vi "DaNISim.vi"(4 "Sonar offset angle":dbl, 5 "Action":enum16{"Init", "Run", "Release"}(ring), 6 "Sonar angle":dbl, 7 "Mode Select":T1(ring), 8 "error in (no error)":errorcluster, 9 "IP Adress":T2, 10 "Ul":dbl, 11 "Ur":dbl) -> (0 "error out":errorcluster, 1 "Sonar distance":fxp<+,32,8>, 2 "OmegaL":dbl, 3 "OmegaR":dbl)   [LabVIEW 2016]
uses:
  <vilib>/userdefined/High Color/nirio_resource_hc.ctl
  <vilib>/FPGAPlugInAG/sbRIO-9632/niLvFpga_Open_sbRIO-9632.vi
  <vilib>/rvi/interface/common/dynamic/niFpgaDynamicAddResources.vi
  <vilib>/Utility/error.llb/Error Cluster From Error Code.vi
  <vilib>/rvi/errors/niLvFpgaAdjustHostInterfaceError.vi
  <vilib>/FPGAPlugInAG/Dynamic/niLvFpga_Close_Dynamic.vi
  <vilib>/rvi/interface/nirviOpenFPGA/nirviOpenFPGA.xnode
  FPGA Bitfiles/StarterKit2.0Cus_FPGATarget_StarterKit2.0Cus_pLn805qeh78.lvbitx
  <vilib>/rvi/interface/nirviReadWriteControl/nirviReadWriteControl.xnode
  <vilib>/rvi/interface/nirviCloseFPGA/nirviCloseFPGA.xnode
  NiFpgaLv.dll
  <vilib>/rvi/interface/Simulation/niFpgaSimulationCallBeginRW.vi
panel:
  in  "N":i32=100
  in  "J":dbl=0.03
  in  "L":dbl=0.1825
  in  "R":dbl=0.046
  in  "M":dbl=3.0
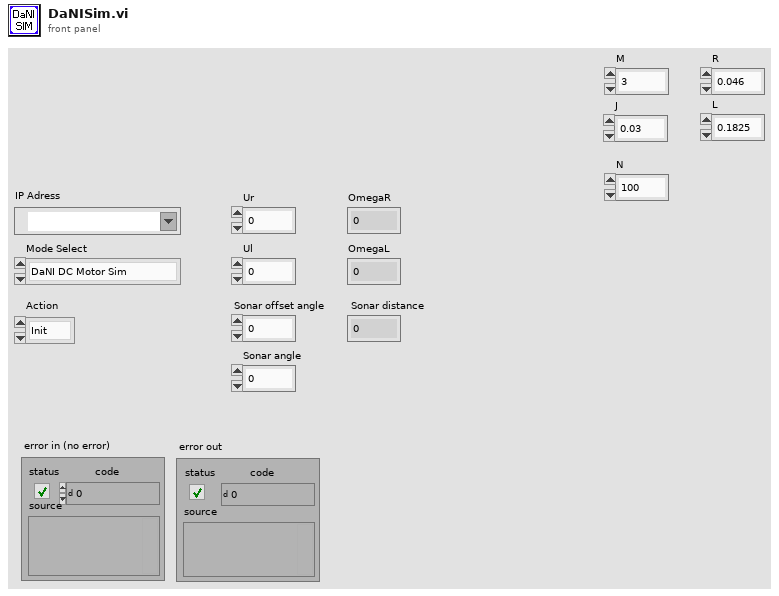
[diagram p1: front panel]
types:
  T1 = enum16{"DaNI DC Motor Sim", "DaNI Simulation", "DaNI Robot"}
  T2 = typedef "nirio_resource_hc.ctl" = tag
  T3 = cluster{"period (uSec)":u32, "pulse width (uSec)":u32}
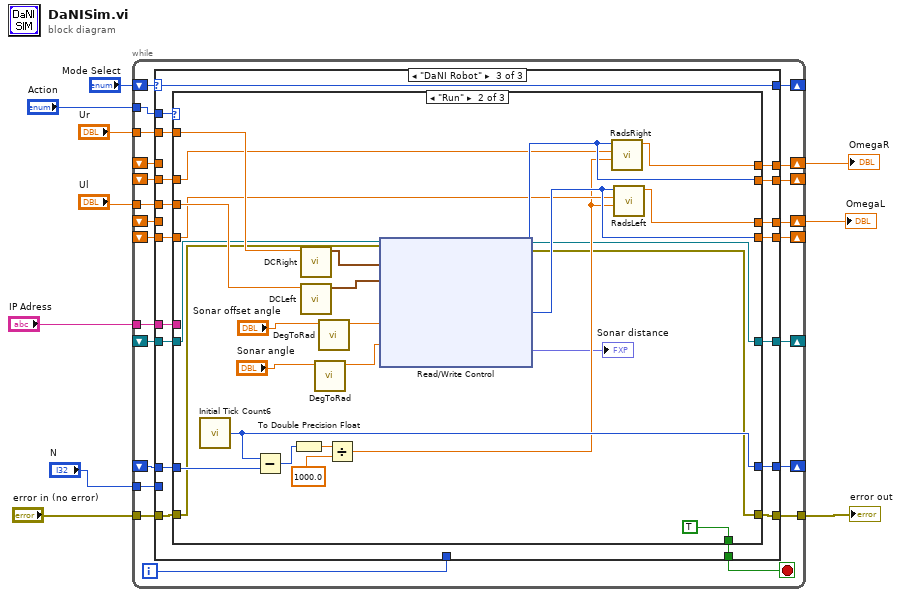
[diagram p0: block diagram]
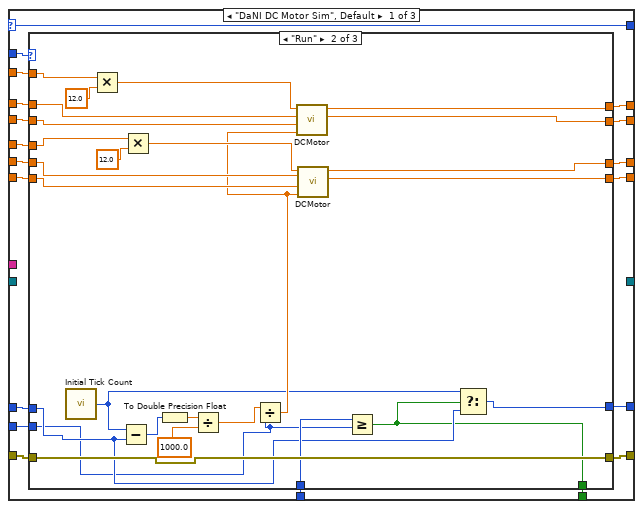
[diagram p2: hidden frame]
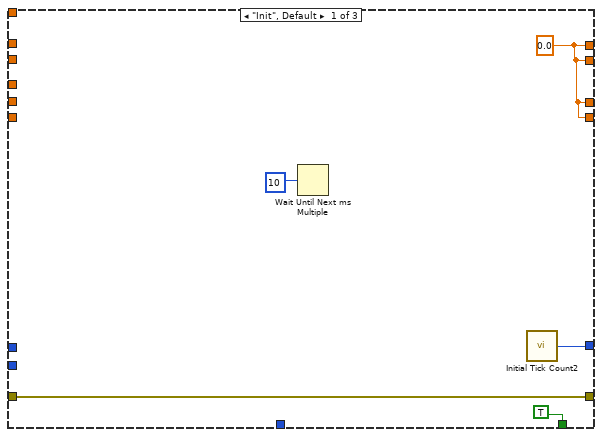
[diagram p3: hidden frame]
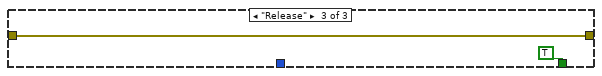
[diagram p4: hidden frame]
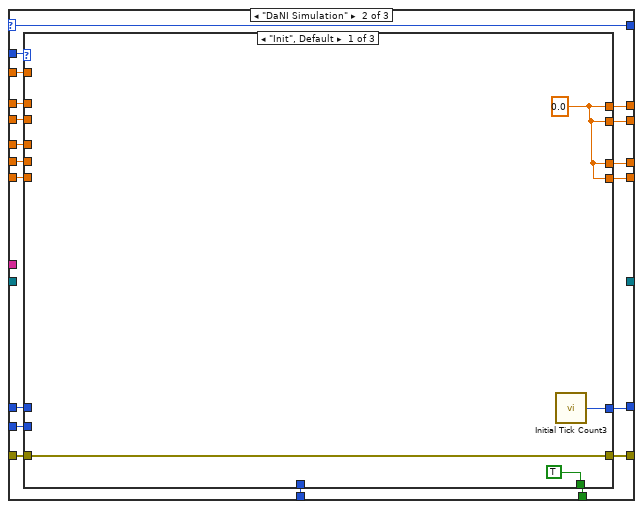
[diagram p5: hidden frame]
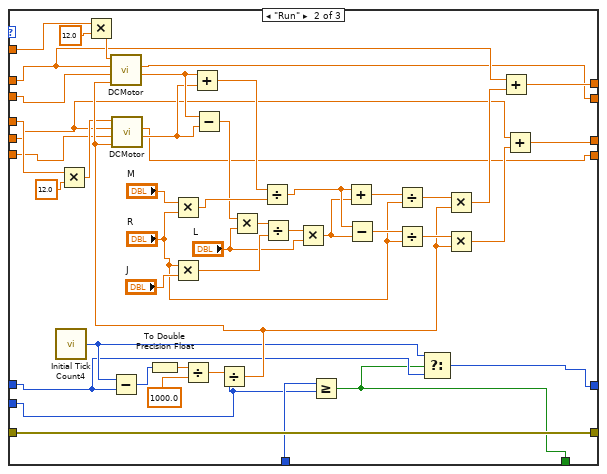
[diagram p6: hidden frame]
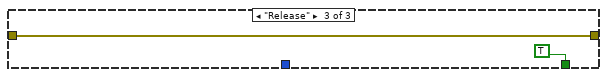
[diagram p7: hidden frame]
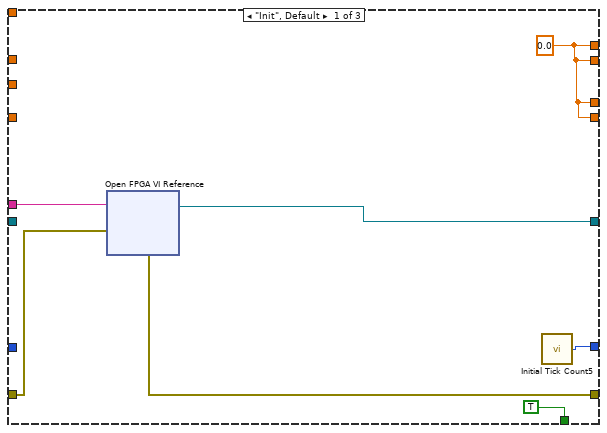
[diagram p8: hidden frame]
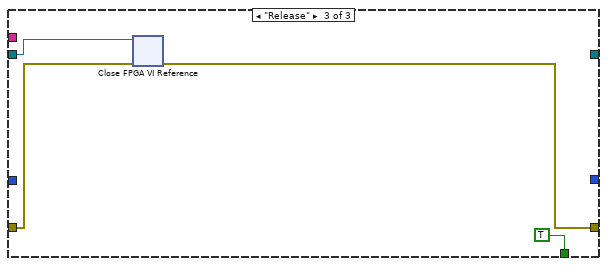
[diagram p9: hidden frame]
diagram:
  n1 = while {
    shift-right: [w31] -> w4
    shift-left: _ -> [w22]
    shift-right: [w30] -> _
    shift-left: _ -> [w21]
    tunnel: "Ur" -> [w23]
    tunnel: "error in (no error)" -> [w27]
    shift-right: [w29] -> w3
    shift-left: _ -> [w19]
    shift-right: [w28] -> _
    shift-left: _ -> [w18]
    tunnel: "Ul" -> [w20]
    shift-right: [w24] -> _
    shift-left: _ -> [w25]
    shift-right: [w14] -> _
    shift-left: _ -> [w13]
    tunnel: "IP Adress" -> [w15]
    tunnel: "Action" -> [w32]
    tunnel: [w26] -> w2
    shift-right: [w12] -> _
    shift-left: "Mode Select" -> [w33]
    tunnel: "N" -> [w11]
    i -> [w16]
    stop <- w17 stop-if-true
    n2 = case shown="\"DaNI Robot\"" w33 {
      selector: w33 -> [w36 w87 w157]
      tunnel: w32 -> [w52 w100 w168]
      tunnel: [w51 w104 w174] -> w31
      tunnel: [w50 w103 w173] -> w30
      tunnel: [w49 w102 w172] -> w29
      tunnel: [w48 w101 w171] -> w28
      tunnel: w27 -> [w39 w98 w170]
      tunnel: [w38 w97 w169] -> w26
      tunnel: w25 -> [w47 w89 w160]
      tunnel: [w46 w96 w167] -> w24
      tunnel: w23 -> [w45 w95 w164]
      tunnel: w22 -> [w44 w94 _]
      tunnel: w21 -> [w43 w93 w162]
      tunnel: w20 -> [w42 w92 w163]
      tunnel: w19 -> [w41 w90 _]
      tunnel: w18 -> [w40 w91 w161]
      tunnel: [w37 w99 w158] -> w17
      tunnel: w16 -> [w35 w88 _]
      tunnel: w15 -> [_ _ w166]
      tunnel: [_ _ w165] -> w14
      tunnel: w13 -> [_ _ w159]
      tunnel: [w36 w87 w157] -> w12
      tunnel: w11 -> [w34 w86 _]
      frame "DaNI DC Motor Sim", Default {
        n3 = case shown="\"Run\"" w52 {
          tunnel: [w57 w70 _] -> w51
          tunnel: [w57 w69 _] -> w50
          tunnel: [w57 w68 _] -> w49
          tunnel: [w57 w67 _] -> w48
          tunnel: w47 -> [_ w61 _]
          tunnel: [w54 w59 _] -> w46
          tunnel: w45 -> [_ w76 _]
          tunnel: w44 -> [_ w75 _]
          tunnel: w43 -> [_ w74 _]
          tunnel: w42 -> [_ w73 _]
          tunnel: w41 -> [_ w72 _]
          tunnel: w40 -> [_ w71 _]
          tunnel: w39 -> [w55 w66 w85]
          tunnel: [w55 w66 w85] -> w38
          tunnel: [TRUE w60 TRUE] -> w37
          tunnel: w35 -> [_ w63 _]
          tunnel: w34 -> [_ w58 _]
          frame "Init", Default {
            w57 = 0.0
            n4 = Wait Until Next ms Multiple(millisecond multiple=u32 10) -> ()  [unwired: 1 out]
            n5 = call "Initial Tick Count2"() -> ("Tick Count(mSec)"=w54:u32)
          }
          frame "Run" {
            n6 = call "Initial Tick Count"() -> ("Tick Count(mSec)"=w62:u32)
            n7 = Multiply(x=w76, y=12.0) -> (x*y=w79:dbl)
            n8 = Subtract(x=w62, y=w61) -> (x-y=w83:u32)
            n9 = Multiply(x=w73, y=12.0) -> (x*y=w77:dbl)
            n10 = To Double Precision Float(number=w83) -> (double precision float=w81:dbl)
            n11 = Divide(x=w81, y=1000.0) -> (x/y=w65:dbl)
            n12 = Divide(x=w65, y=w58) -> (x/y=w64:dbl)
            n13 = call "DCMotor.vi"("dt"=w64, "I"=w74, "Omega"=w75, "V"=w79) -> ("I Out"=w69:dbl, "Omega Out"=w70:dbl)  [unwired: 5 in, 1 out]
            n14 = call "DCMotor.vi"("dt"=w64, "I"=w71, "Omega"=w72, "V"=w77) -> ("I Out"=w67:dbl, "Omega Out"=w68:dbl)  [unwired: 5 in, 1 out]
            n15 = Greater Or Equal?(x=w63, y=w58) -> (x >= y?=w60:bool)
            n16 = Select(t=w62, s=w60, f=w61) -> (s? t:f=w59:u32)
          }
          frame "Release" {
          }
        }
      }
      frame "DaNI Simulation" {
        n17 = case shown="\"Init\", Default" w100 {
          tunnel: [w108 w117 _] -> w104
          tunnel: [w108 w115 _] -> w103
          tunnel: [w108 w116 _] -> w102
          tunnel: [w108 w114 _] -> w101
          tunnel: [TRUE w111 TRUE] -> w99
          tunnel: w98 -> [w106 w154 w156]
          tunnel: [w106 w154 w156] -> w97
          tunnel: [w105 w112 _] -> w96
          tunnel: w95 -> [_ w123 _]
          tunnel: w94 -> [_ w122 _]
          tunnel: w93 -> [_ w121 _]
          tunnel: w92 -> [_ w120 _]
          tunnel: w91 -> [_ w119 _]
          tunnel: w90 -> [_ w118 _]
          tunnel: w89 -> [_ w113 _]
          tunnel: w88 -> [_ w110 _]
          tunnel: w86 -> [_ w109 _]
          frame "Init", Default {
            w108 = 0.0
            n18 = call "Initial Tick Count3"() -> ("Tick Count(mSec)"=w105:u32)
          }
          frame "Run" {
            n19 = call "Initial Tick Count4"() -> ("Tick Count(mSec)"=w128:u32)
            n20 = Multiply(x=w120, y=12.0) -> (x*y=w124:dbl)
            n21 = Multiply(x=w123, y=12.0) -> (x*y=w126:dbl)
            n22 = Subtract(x=w128, y=w113) -> (x-y=w151:u32)
            n23 = To Double Precision Float(number=w151) -> (double precision float=w153:dbl)
            n24 = Multiply(x="M", y="R") -> (x*y=w145:dbl)
            n25 = Multiply(x="R", y="J") -> (x*y=w142:dbl)
            n26 = Divide(x=w153, y=1000.0) -> (x/y=w130:dbl)
            n27 = Divide(x=w130, y=w109) -> (x/y=w129:dbl)
            n28 = call "DCMotor.vi"("dt"=w129, "I"=w121, "Omega"=w122, "V"=w126) -> ("Torque Out"=w148:dbl, "I Out"=w115:dbl)  [unwired: 5 in, 1 out]
            n29 = call "DCMotor.vi"("dt"=w129, "I"=w119, "Omega"=w118, "V"=w124) -> ("Torque Out"=w147:dbl, "I Out"=w114:dbl)  [unwired: 5 in, 1 out]
            n30 = Add(x=w148, y=w147) -> (x+y=w146:dbl)
            n31 = Subtract(x=w148, y=w147) -> (x-y=w144:dbl)
            n32 = Multiply(x=w144, y="L") -> (x*y=w143:dbl)
            n33 = Divide(x=w146, y=w145) -> (x/y=w139:dbl)
            n34 = Divide(x=w143, y=w142) -> (x/y=w141:dbl)
            n35 = Multiply(x=w141, y="L") -> (x*y=w138:dbl)
            n36 = Greater Or Equal?(x=w110, y=w109) -> (x >= y?=w111:bool)
            n37 = Add(x=w139, y=w138) -> (x+y=w137:dbl)
            n38 = Subtract(x=w139, y=w138) -> (x-y=w136:dbl)
            n39 = Divide(x=w137, y="R") -> (x/y=w134:dbl)
            n40 = Divide(x=w136, y="R") -> (x/y=w133:dbl)
            n41 = Select(t=w128, s=w111, f=w113) -> (s? t:f=w112:u32)
            n42 = Multiply(x=w134, y=w129) -> (x*y=w132:dbl)
            n43 = Multiply(x=w133, y=w129) -> (x*y=w131:dbl)
            n44 = Add(x=w122, y=w132) -> (x+y=w117:dbl)
            n45 = Add(x=w118, y=w131) -> (x+y=w116:dbl)
          }
          frame "Release" {
          }
        }
      }
      frame "DaNI Robot" {
        n46 = case shown="\"Run\"" w168 {
          tunnel: [w181 w203 _] -> w174
          tunnel: [w181 w202 _] -> w173
          tunnel: [w181 w201 _] -> w172
          tunnel: [w181 w200 _] -> w171
          tunnel: w170 -> [w177 w190 w209]
          tunnel: [w176 w189 w208] -> w169
          tunnel: [w180 w193 _] -> w167
          tunnel: w166 -> [w179 _ _]
          tunnel: [w178 w188 _] -> w165
          tunnel: w164 -> [_ w205 _]
          tunnel: w163 -> [_ w204 _]
          tunnel: w162 -> [_ w199 _]
          tunnel: w161 -> [_ w198 _]
          tunnel: w160 -> [_ w194 _]
          tunnel: w159 -> [_ w191 w210]
          tunnel: [TRUE TRUE TRUE] -> w158
          frame "Init", Default {
            w181 = 0.0
            n47 = xnode "Open FPGA VI Reference"("error in"=w177, "resource name"=w179) -> ("FPGA VI Reference Out"=w178:refnum<k20>, "error out"=w176:errorcluster)
            n48 = call "Initial Tick Count5"() -> ("Tick Count(mSec)"=w180:u32)
          }
          frame "Run" {
            n49 = call "Initial Tick Count6"() -> ("Tick Count(mSec)"=w193:u32)
            n50 = Subtract(x=w193, y=w194) -> (x-y=w197:u32)
            n51 = To Double Precision Float(number=w197) -> (double precision float=w195:dbl)
            n52 = call "DCRight.vi"("Dc In"=w205) -> ("PWM Right Motor"=w207:T3)  [unwired: 10 in]
            n53 = call "DCLeft.vi"("Dc In"=w204) -> ("PWM Left Motor"=w206:T3)  [unwired: 10 in]
            n54 = call "DegToRad.vi"("Degrees"="Sonar angle") -> ("Radians"=w182:dbl)  [unwired: 10 in]
            n55 = call "DegToRad.vi"("Degrees"="Sonar offset angle") -> ("Radians"=w185:dbl)  [unwired: 10 in]
            n56 = Divide(x=w195, y=1000.0) -> (x/y=w192:dbl)
            n57 = xnode "Read/Write Control"("FPGA VI Reference In"=w191, "error in"=w190, "PWM Right Motor"=w207, "PWM Left Motor"=w206, "hs400_0_ccw offset"=w185, "hs400_0_ccw angle"=w182) -> ("FPGA VI Reference Out"=w188:refnum<k20>, "error out"=w189:errorcluster, "Right cw count (pulses)"=w202:i32, "Left cw count (pulses)"=w200:i32, "PING)))_0_dist"=→"Sonar distance":fxp<+,32,8>)
            n58 = call "RadsRight.vi"("dt"=w192, "Cw2"=w199, "Cw1"=w202) -> ("Rs"=w203:dbl)  [unwired: 8 in]
            n59 = call "RadsLeft.vi"("dt"=w192, "Cw2"=w198, "Cw1"=w200) -> ("Rs"=w201:dbl)  [unwired: 8 in]
          }
          frame "Release" {
            n60 = xnode "Close FPGA VI Reference"("FPGA VI Reference In"=w210, "error in"=w209) -> ("error out"=w208:errorcluster)
          }
        }
      }
    }
  }
  "OmegaR" <- w4
  "error out" <- w2
  "OmegaL" <- w3
